vi "Wait Socket (Socket).vi"(8 "error in (no error)":errorcluster, 9 "timeout ms (25000)":u32=25000, 10 "socket":u64, 11 "session":T1) -> (0 "error out":errorcluster)   [LabVIEW 2017, in "libssh2.lvlib"]
doc: "Wait for data on a TCP socket in reading or writing direction as indicated by the session."
uses:
  libssh2.lvlib
  Session Refnum.ctl
  libssh2_session_block_direction.ctl
  Not A Session.vi
  Ws2_32.dll
  libc.so.6
panel:
  out "return type":i32
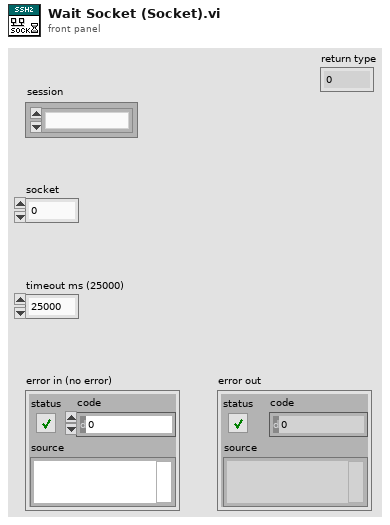
[diagram p1: front panel]
types:
  T1 = typedef "libssh2.lvlib/Session Refnum.ctl" = refnum<k1>
  T2 = typedef "libssh2.lvlib/libssh2_session_block_direction.ctl" = i32
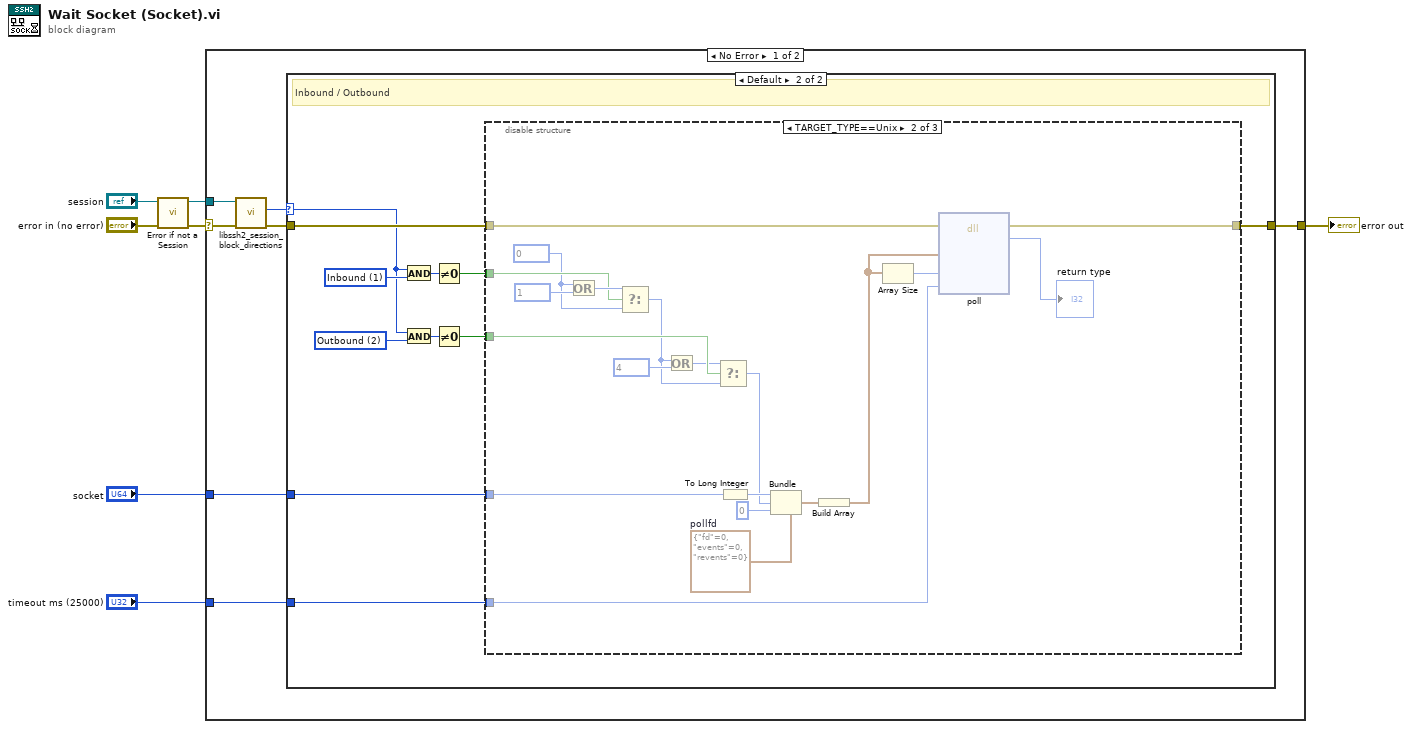
[diagram p0: block diagram]
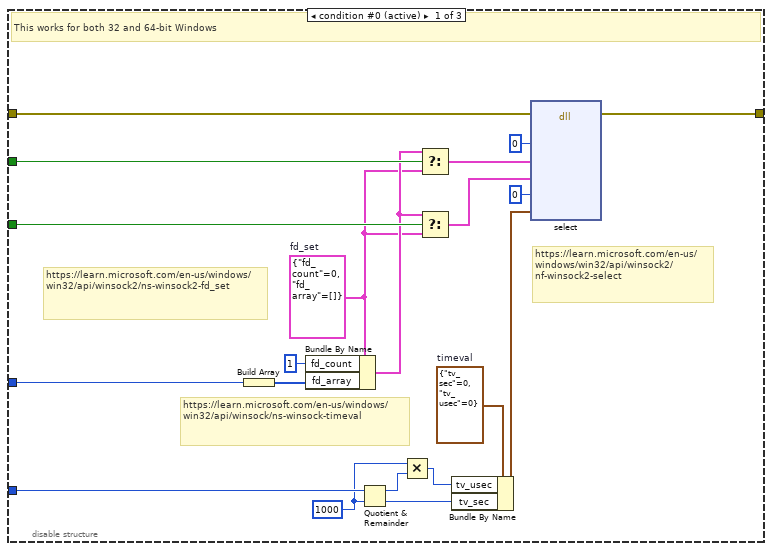
[diagram p3: hidden frame]
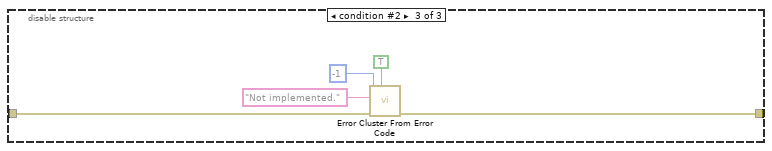
[diagram p4: hidden frame]
diagram:
  n1 = call "Error if not a Session.vi"("error in (no error)"="error in (no error)", "session"="session") -> ("error out"=w2:errorcluster, "session out"=w3:T1)  [unwired: 8 in]
  n2 = case shown="No Error" w2 {
    selector: w2 -> [w10 w72]
    tunnel: [w14 w72] -> w6
    tunnel: "socket" -> [w13 _]
    tunnel: w3 -> [w11 _]
    tunnel: "timeout ms (25000)" -> [w9 _]
    frame No Error {
      n3 = call "libssh2_session_block_directions.vi"("error in (no error)"=w10, "session"=w11) -> ("error out"=w12:errorcluster, "block direction"=w8:T2)  [unwired: 8 in]
      n4 = case shown="Default" w8 {
        selector: w8 -> [_ w16]
        tunnel: [w15 w26] -> w14
        tunnel: w13 -> [_ w25]
        tunnel: w12 -> [w15 w24]
        tunnel: w9 -> [_ w17]
        frame 0 {
          # "None"
        }
        frame Default {
          w23 = T2 2 items=["Inbound"=1, "Outbound"=2] ("block direction")
          w22 = T2 1 items=["Inbound"=1, "Outbound"=2] ("block direction")
          # "Inbound / Outbound"
          n5 = And(x=w16, y=w22) -> (x .and. y?=w21:T2)
          n6 = And(x=w16, y=w23) -> (x .and. y?=w20:T2)
          n7 = Not Equal To 0?(x=w21) -> (x != 0?=w19:bool)
          n8 = Not Equal To 0?(x=w20) -> (x != 0?=w18:bool)
          n9 = disable-structure shown="TARGET_TYPE==Unix" {
            disable-tunnel: [w43 w62 w70] -> w26
            disable-tunnel: w25 -> [w42 w66 _]
            disable-tunnel: w24 -> [w41 w63 w71]
            disable-tunnel: w19 -> [w40 w57 _]
            disable-tunnel: w18 -> [w38 w56 _]
            disable-tunnel: w17 -> [w33 w64 _]
            frame condition #0 (active) {
              w29 = u32 1000 ("y")
              w36 = cluster{"fd_count":u32, "fd_array":u32[]} {"fd_count"=0, "fd_array"=[]}  # fd_set
              w35 = cluster{"tv_sec":u32, "tv_usec":u32} {"tv_sec"=0, "tv_usec"=0}  # timeval
              # "https://learn.microsoft.com/en-us/windows/win32/api/winsock/ns-winsock-timeval"
              # "https://learn.microsoft.com/en-us/windows/win32/api/winsock2/nf-winsock2-select"
              # "https://learn.microsoft.com/en-us/windows/win32/api/winsock2/ns-winsock2-fd_set"
              # "This works for both 32 and 64-bit Windows"
              n10 = Build Array(w42) -> (w45:u64[])
              n11 = Bundle By Name(cluster=w36, "fd_count"=u32 1, "fd_array"=w45) -> (w37:cluster{"fd_count":u32, "fd_array":u32[]})
              n12 = Quotient & Remainder(x=w33, y=w29) -> (x-y*floor(x/y)=w31:u32, floor(x/y)=w32:u32)
              n13 = Multiply(x=w29, y=w31) -> (x*y=w30:u32)
              n14 = Select(t=w37, s=w40, f=w36) -> (s? t:f=w39:cluster{"fd_count":u32, "fd_array":u32[]})
              n15 = Select(t=w37, s=w38, f=w36) -> (s? t:f=w27:cluster{"fd_count":u32, "fd_array":u32[]})
              n16 = Bundle By Name(cluster=w35, "tv_usec"=w30, "tv_sec"=w32) -> (w34:cluster{"tv_sec":u32, "tv_usec":u32})
              n17 = dll-call lib="Ws2_32.dll" fn="select"(error in=w41, "nfds"=0, "readfds"=w39, "writefds"=w27, "exceptfds"=u32 0 ("nfds"), "timeout"=w34) -> (error out=w43:errorcluster)  [unwired: 8 in, 1 out]
            }
            frame condition #1 {
              w49 = cluster{"fd":i32, "events":u16, "revents":u16} {"fd"=0, "events"=0, "revents"=0}  # pollfd
              w53 = u16 0
              n18 = Or(x=w53, y=u16 1) -> (x .or. y?=w58:u16)
              n19 = Select(t=w58, s=w57, f=w53) -> (s? t:f=w52:u16)
              n20 = Or(x=w52, y=u16 4) -> (x .or. y?=w54:u16)
              n21 = Select(t=w54, s=w56, f=w52) -> (s? t:f=w48:u16)
              n22 = To Long Integer(number=w66) -> (32bit integer=w51:i32)
              n23 = Bundle(cluster=w49, "fd"=w51, "events"=w48, "revents"=u16 0) -> (w65:cluster{"fd":i32, "events":u16, "revents":u16})
              n24 = Build Array(w65) -> (w60:cluster{"fd":i32, "events":u16, "revents":u16}[])
              n25 = Array Size(array=w60) -> (size(s)=w61:i32)
              n26 = dll-call lib="libc.so.6" fn="poll"(error in=w63, "fds"=w60, "nfds"=w61, "timeout"=w64) -> (error out=w62:errorcluster, "return type"=→"return type":i32)  [unwired: 5 in, 1 out]
            }
            frame condition #2 {
              n27 = call <vilib>:"Error Cluster From Error Code.vi"("show call chain? (False)"=TRUE, "error in (no error)"=w71, "error message (\"\")"="Not implemented." ("error message (\"\")"), "error code (0)"=-1) -> ("error out"=w70:errorcluster)  [unwired: 5 in]
            }
          }
        }
      }
    }
    frame Error {
    }
  }
  "error out" <- w6
